vi "_RSA_PKCS1.vi"() -> ()   [LabVIEW 2023]
panel:
  out "tick":u32
  in  "Tab Control":enum32{"密钥生成", "加密解密"}(tab)
  in  "生成秘钥":bool
  in  "填入密钥":bool
  out "公钥":string
  out "私钥":string
  out "?":string
  in  "密钥位数":string(combo)="308"
  in  "原文":string="天空有着多少颗的星辰\n地上就有多少段的人生\n外头无论多么样的寒冷\n蜂蜜酒能把我们给捂热\n欢迎各位光临星河旅馆！"
  out "密文":string
  in  "密文":string
  out "原文":string
  in  "加密":bool
  in  "解密":bool
  in  "公钥":string="-----BEGIN RSA PUBLIC KEY-----\nMIIBCgKCAQECJTwZ2lRcKrdTU5zbP4z6rGr57lWznUWXeU/0eLCZ14Efdue8kDYj\ncuNkpjTIbWBGzZMtdoRwx8lVMC5QrfBdp8Z0nIlqdQvrehlQ/IY9xlbD70XQugy0\nvE1Zmccf/ex+oCsI7Rl1+JaAEsmBIPdWX6dpDelnwkPRapSc2BAyo8R3d6naFasE\nK+y4iqP5SAZjpi9/uEQ9JqqLm8QMkNIqmiqWLyoRZkTEwvw76ODYCu/k+xfulWsh\nC2aG7vTpwTCx7sU7E38QPgA/ICCj2U98wi4VcYiLVVyEXuDKF5WR4FKpMV93n8rY\nw8Kw5xqqdEjMKdE0ARgj7lb3hH9wmUEYlQIDAQAB\n-----END RSA PUBLIC KEY-----"
  in  "私钥":string="-----BEGIN RSA PRIVATE KEY-----\nMIIEpgIBAAKCAQECJTwZ2lRcKrdTU5zbP4z6rGr57lWznUWXeU/0eLCZ14Efdue8\nkDYjcuNkpjTIbWBGzZMtdoRwx8lVMC5QrfBdp8Z0nIlqdQvrehlQ/IY9xlbD70XQ\nugy0vE1Zmccf/ex+oCsI7Rl1+JaAEsmBIPdWX6dpDelnwkPRapSc2BAyo8R3d6na\nFasEK+y4iqP5SAZjpi9/uEQ9JqqLm8QMkNIqmiqWLyoRZkTEwvw76ODYCu/k+xfu\nlWshC2aG7vTpwTCx7sU7E38QPgA/ICCj2U98wi4VcYiLVVyEXuDKF5WR4FKpMV93\nn8rYw8Kw5xqqdEjMKdE0ARgj7lb3hH9wmUEYlQIDAQABAoIBAQIBlYDLU2VYIFOP\n9TZj582kGuiZQJSTtTaenvCJRwKkrT6h7rK525YsYYyFiwf8lzG+HClAETpw58h8\nJGMXM5QwRfhXRHxC9SF97Fx5toHfjNTtUsiKoUUEbAQkMzqsNFB4L6XKKKvTB9C9\nQKY6EG85RQ+MjbyTwNz7n/pGZGcmDlPM7dlFwKN5LxS931CcjIC8FcXqCb2hfPIn\nR7L4hmbvT8vSZe3LfwSMcIu3dbL7Uh1N1URtDSiFu785GYtl2WLHTrTE2F38ygYe\nY7KJ5kLNr91ULJfUatukeSolfndqnlWPisoshtopYisDeL+2olHjvl0VGk8j1t5c\nU6PAL3fhAoGBBAq9XeIIIMu9gYEY4rCES++Y1u+SGp/ET/e0aFEq9a5aiZdce9m/\nEaUsd+suffk3sqabG9Mb8SaNremsMpptrxtwVnaLlr6OZxQV2KaT+3AFI1m8Vs6d\n8IFQdD5/62XIXVCRQgUJyZwxcHY6uNZ5KwLpQ7VgTNLWFys3PnP9/wVdAoGBAIfi\nMAnVVHpeAgXo3hOd5/1FapFC0yH2tJv7VcHjd9r++0JC2xCEnLJ4P1jHHOK0sJ+W\nCHRXiY2q6ihiMtue3LbE8KQTJ4gECf6LqrEdijw8KwyQclCOhdtdtOG31gfQIlxH\n+L8lnha2Gln2kYuIHS/EnTb2v+2nCf9LM+lNwDSZAoGBAsbeEgGXU/Ck4LOwRQy/\n1utkNUWhOmlIlSe36XLZ8K83xA8Ymn2dpqGzSy9nYWQ1v6Z2KUd/iszRyQkgJCOz\n9vkC1GPcwlNnwakq2QyX3cW3wfGEUp7gIrq0aygE+dOTM4iGQrTzZG7KCFkxPosZ\n81KsrreM0TqHmqM18NH/TZSBAoGBAIYOCJR66Ne8DMTlwsmZm/hK1mKuiXrVV8MW\nxrj8fw8HRLxPFq2KFskfRmeAMCgcWK9oJbkZbzPbLR1gG4p9hIOvcTR9TR+r1GxS\nP7hySyE3vsSrcIu2v6n2HXAdnEKi/HML8gQpyXfgecjNLzN3ukuY7fz+m8SKaZt6\nBqGhOgDpAoGBAw/yVr0DlLIgLzbeIWyrIeXSE8C7c/wH1fnUlt+sILGcUZIdUR9H\nLNTdImxRtSZFOgwS7V2hT3S6X4+SavwKWLRs0Bq1ZbHVCBsx7WotmtYb8MPyJChP\nkkSuCOkYuEU5yGVSwSNHa2QpbnpoM2wGuaBAD3qGTQ4EoO4vr/4kEJqZ\n-----END RSA PRIVATE KEY-----"
  in  "填入密文":bool
  out "加解密提示":string
  in  "填入密钥":bool
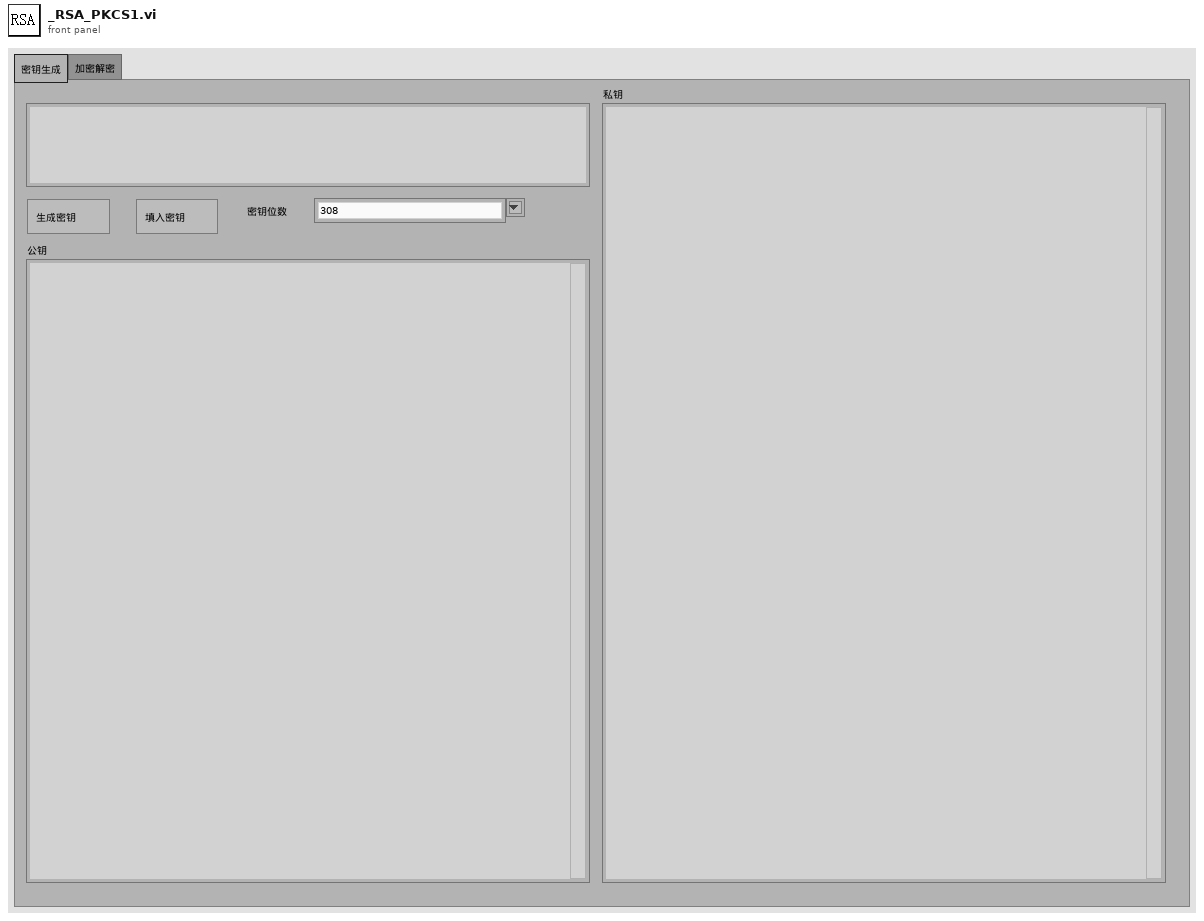
[diagram p1: front panel]
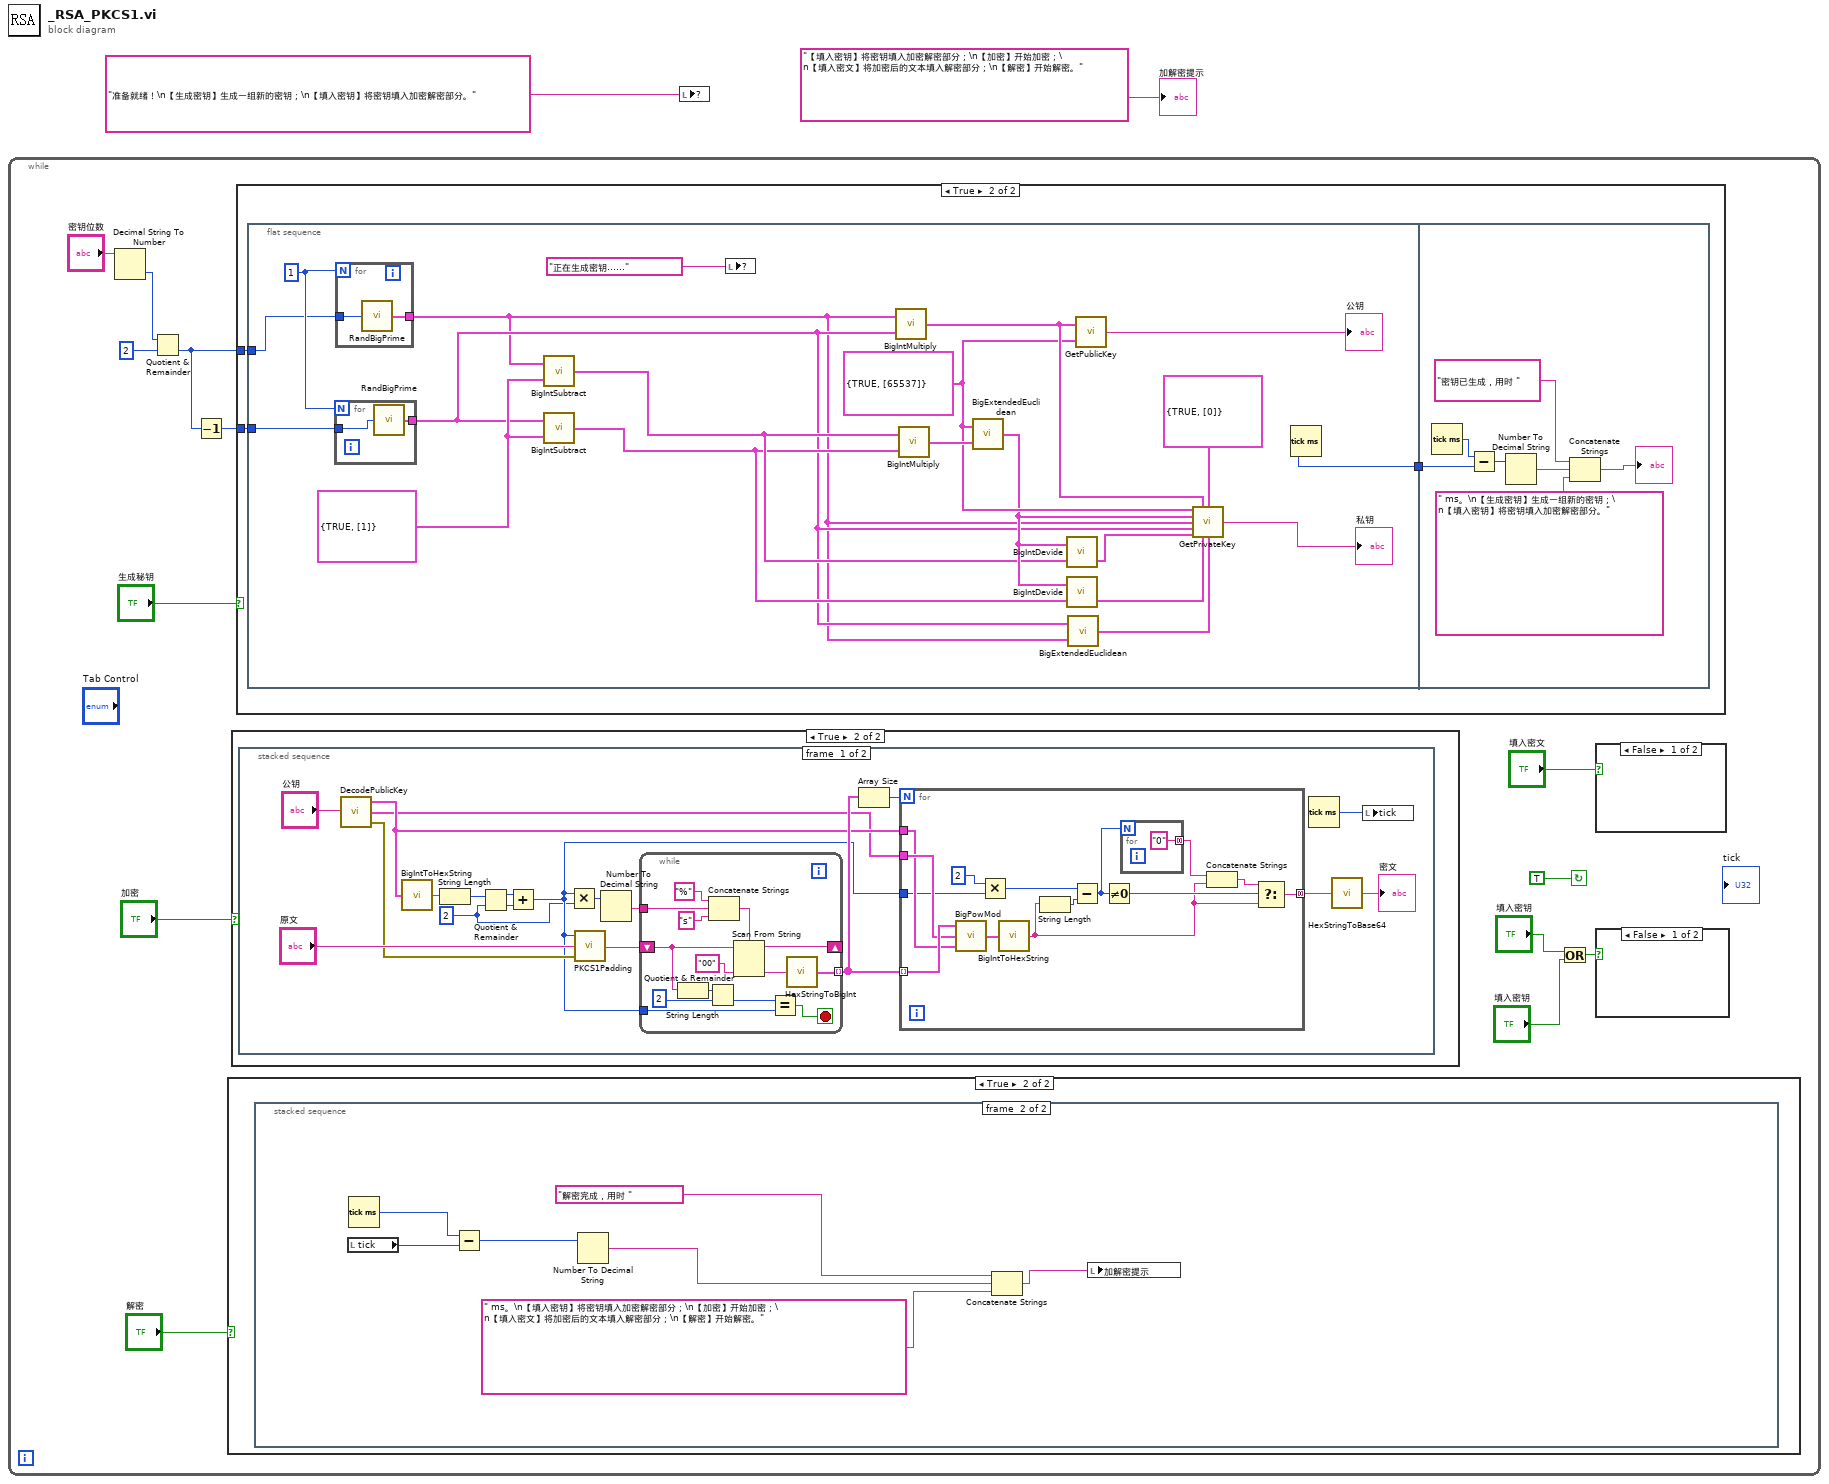
[diagram p0: block diagram]
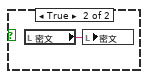
[diagram p2: hidden frame]
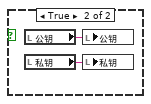
[diagram p3: hidden frame]
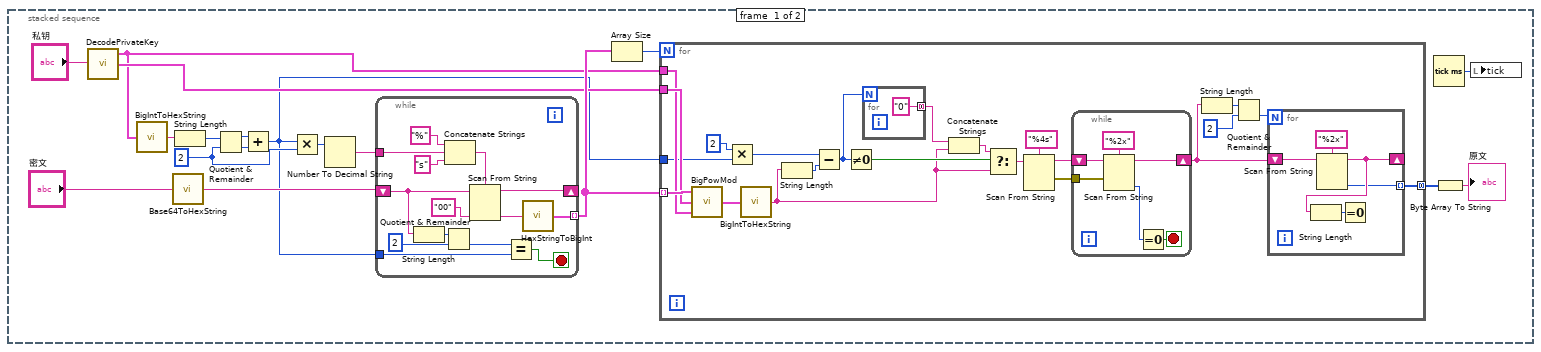
[diagram p5: hidden frame]
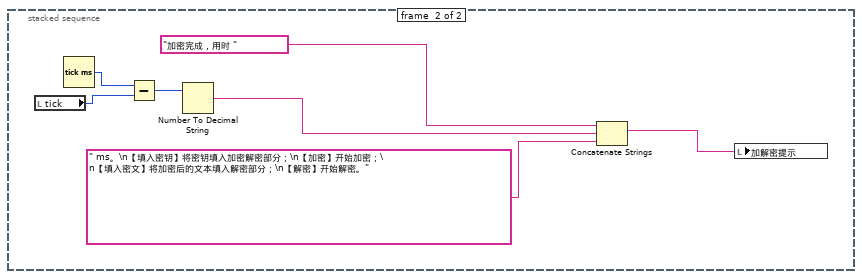
[diagram p7: hidden frame]
diagram:
  n1 = while {
    stop <- TRUE continue-if-true
    n2 = Decimal String To Number(string="密钥位数") -> (number=w8:i32)  [unwired: 2 in, 1 out]
    n3 = Quotient & Remainder(x=w8, y=2) -> (floor(x/y)=w7:i32)  [unwired: 1 out]
    n4 = Decrement(x=w7) -> (x-1=w6:i32)
    n5 = case shown="True" "解密" {
      frame False {
      }
      frame True {
        n6 = stacked-sequence {
          frame #0 {
            w31 = 2
            n7 = call "DecodePrivateKey.vi"("Private Key"="私钥") -> ("d"=w24:cluster{"P/N":bool, "Array":u64[]}, "n"=w23:cluster{"P/N":bool, "Array":u64[]})  [unwired: 2 in, 1 out]
            n8 = call "BigIntToHexString.vi"("a"=w23) -> ("Hex string"=w35:string)
            n9 = call "Base64ToHexString.vi"("BASE64 string"="密文") -> ("Hex"=w27:string)
            n10 = String Length(string=w35) -> (length=w34:i32)
            n11 = Quotient & Remainder(x=w34, y=w31) -> (x-y*floor(x/y)=w33:i32, floor(x/y)=w32:i32)
            n12 = Add(x=w33, y=w32) -> (x+y=w22:i32)
            n13 = Multiply(x=w22, y=w31) -> (x*y=w30:i32)
            n14 = Number To Decimal String(number=w30) -> (decimal integer string=w29:string)  [unwired: 1 in]
            n15 = while {
              tunnel: w29 -> [w83]
              tunnel: w22 -> [w78]
              shift-right: [w75] -> _
              shift-left: w27 -> [w77]
              tunnel: [w74] -> w25 mode=indexing
              stop <- w76 stop-if-true
              n16 = String Length(string=w77) -> (length=w72:i32)
              n17 = Quotient & Remainder(x=w72, y=2) -> (floor(x/y)=w73:i32)  [unwired: 1 out]
              n18 = Concatenate Strings("%", w83, "s") -> (w81:string)
              n19 = Scan From String(format string=w81, input string=w77, default 1="00") -> (remaining string=w75:string, output 1=w79:string)  [unwired: 2 in, 2 out]
              n20 = Equal?(x=w73, y=w78) -> (x = y?=w76:bool)
              n21 = call "HexStringToBigInt.vi"("String (hex)"=w79) -> ("Int"=w74:cluster{"P/N":bool, "Array":u64[]})
            }
            n22 = Array Size(array=w25) -> (size(s)=w26:i32)
            n23 = for {
              N: w26 -> [_]
              tunnel: w25 -> [w58] mode=indexing
              tunnel: w24 -> [w57]
              tunnel: w23 -> [w56]
              tunnel: w22 -> [w43]
              tunnel: [w41] -> w21 mode=concatenating
              n24 = call "BigPowMod.vi"("c"=w56, "b"=w57, "a"=w58) -> ("a ^ b mod c"=w49:cluster{"Boolean":bool, "Array":u64[]})
              n25 = Multiply(x=2, y=w43) -> (x*y=w47:i32)
              n26 = call "BigIntToHexString.vi"("a"=w49) -> ("Hex string"=w51:string)
              n27 = String Length(string=w51) -> (length=w55:i32)
              n28 = Subtract(x=w47, y=w55) -> (x-y=w53:i32)
              n29 = Not Equal To 0?(x=w53) -> (x != 0?=w54:bool)
              n30 = for {
                N: w53 -> [_]
                tunnel: ["0"] -> w52 mode=concatenating
              }
              n31 = Concatenate Strings(w52, w51) -> (w50:string)
              n32 = Select(t=w50, s=w54, f=w51) -> (s? t:f=w46:string)
              n33 = Scan From String(format string="%4s", input string=w46) -> (remaining string=w42:string, error out=w44:errorcluster)  [unwired: 4 in, 1 out]
              n34 = while {
                tunnel: w44 -> [w69]
                shift-right: [w64] -> w40
                shift-left: w42 -> [w65]
                stop <- w66 stop-if-true
                n35 = Scan From String(format string="%2x", input string=w65, error in=w69) -> (remaining string=w64:string, output 1=w67:u32)  [unwired: 2 in, 2 out]
                n36 = Equal To 0?(x=w67) -> (x = 0?=w66:bool)
              }
              n37 = String Length(string=w40) -> (length=w38:i32)
              n38 = Quotient & Remainder(x=w38, y=2) -> (floor(x/y)=w39:i32)  [unwired: 1 out]
              n39 = for {
                N: w39 -> [_]
                shift-right: [w61] -> _
                shift-left: w40 -> [w62]
                tunnel: [w59] -> w41 mode=indexing
                n40 = Scan From String(format string="%2x", input string=w62) -> (remaining string=w61:string, output 1=w59:u32)  [unwired: 3 in, 2 out]
                n41 = String Length(string=w61) -> (length=w60:i32)
                n42 = Equal To 0?(x=w60) -> ()  [unwired: 1 out]
              }
            }
            n43 = Tick Count (ms)() -> (millisecond timer value=w19:u32)
            n44 = Byte Array To String(unsigned byte array=w21) -> (string=→"原文":string)
            n45 = local write "tick"(w19) -> ()
          }
          frame #1 {
            n46 = local read "tick"() -> (w85:u32)
            n47 = Tick Count (ms)() -> (millisecond timer value=w86:u32)
            n48 = Subtract(x=w86, y=w85) -> (x-y=w91:u32)
            n49 = Number To Decimal String(number=w91) -> (decimal integer string=w89:string)  [unwired: 1 in]
            n50 = Concatenate Strings("解密完成，用时 ", w89, " ms。\n【填入密钥】将密钥填入加密解密部分；\n【加密】开始加密；\n【填入密文】将加密后的文本填入解密部分；\n【解密】开始解密。") -> (w87:string)
            n51 = local write "加解密提示"(w87) -> ()
          }
        }
      }
    }
    n52 = case shown="True" "加密" {
      frame False {
      }
      frame True {
        n53 = stacked-sequence {
          frame #0 {
            w93 = 2
            n54 = call "DecodePublicKey.vi"("Public Key"="公钥") -> ("error out"=w104:errorcluster, "e"=w98:cluster{"P/N":bool, "Array":u64[]}, "n"=w99:cluster{"P/N":bool, "Array":u64[]})  [unwired: 2 in]
            n55 = call "BigIntToHexString.vi"("a"=w99) -> ("Hex string"=w108:string)
            n56 = String Length(string=w108) -> (length=w107:i32)
            n57 = Quotient & Remainder(x=w107, y=w93) -> (x-y*floor(x/y)=w106:i32, floor(x/y)=w105:i32)
            n58 = Add(x=w106, y=w105) -> (x+y=w97:i32)
            n59 = Multiply(x=w97, y=w93) -> (x*y=w94:i32)
            n60 = call "PKCS1Padding.vi"("error in (no error)"=w104, "Message"="原文", "Length"=w97) -> ("Hex (After Padding)"=w103:string)  [unwired: 1 in, 1 out]
            n61 = Number To Decimal String(number=w94) -> (decimal integer string=w102:string)  [unwired: 1 in]
            n62 = while {
              tunnel: w102 -> [w138]
              tunnel: w97 -> [w133]
              shift-right: [w130] -> _
              shift-left: w103 -> [w132]
              tunnel: [w129] -> w100 mode=indexing
              stop <- w131 stop-if-true
              n63 = String Length(string=w132) -> (length=w127:i32)
              n64 = Quotient & Remainder(x=w127, y=2) -> (floor(x/y)=w128:i32)  [unwired: 1 out]
              n65 = Concatenate Strings("%", w138, "s") -> (w136:string)
              n66 = Scan From String(format string=w136, input string=w132, default 1="00") -> (remaining string=w130:string, output 1=w134:string)  [unwired: 2 in, 2 out]
              n67 = Equal?(x=w128, y=w133) -> (x = y?=w131:bool)
              n68 = call "HexStringToBigInt.vi"("String (hex)"=w134) -> ("Int"=w129:cluster{"P/N":bool, "Array":u64[]})
            }
            n69 = Array Size(array=w100) -> (size(s)=w101:i32)
            n70 = for {
              N: w101 -> [_]
              tunnel: w100 -> [w124] mode=indexing
              tunnel: w99 -> [w122]
              tunnel: w98 -> [w123]
              tunnel: w97 -> [w113]
              tunnel: [w117] -> w95 mode=concatenating
              n71 = call "BigPowMod.vi"("c"=w122, "b"=w123, "a"=w124) -> ("a ^ b mod c"=w121:cluster{"Boolean":bool, "Array":u64[]})
              n72 = Multiply(x=2, y=w113) -> (x*y=w115:i32)
              n73 = call "BigIntToHexString.vi"("a"=w121) -> ("Hex string"=w112:string)
              n74 = String Length(string=w112) -> (length=w120:i32)
              n75 = Subtract(x=w115, y=w120) -> (x-y=w118:i32)
              n76 = Not Equal To 0?(x=w118) -> (x != 0?=w119:bool)
              n77 = for {
                N: w118 -> [_]
                tunnel: ["0"] -> w116 mode=concatenating
              }
              n78 = Concatenate Strings(w116, w112) -> (w111:string)
              n79 = Select(t=w111, s=w119, f=w112) -> (s? t:f=w117:string)
            }
            n80 = Tick Count (ms)() -> (millisecond timer value=w92:u32)
            n81 = call "HexStringToBase64.vi"("Hex"=w95) -> ("BASE64 string"=→"密文":string)
            n82 = local write "tick"(w92) -> ()
          }
          frame #1 {
            n83 = local read "tick"() -> (w140:u32)
            n84 = Tick Count (ms)() -> (millisecond timer value=w141:u32)
            n85 = Subtract(x=w141, y=w140) -> (x-y=w146:u32)
            n86 = Number To Decimal String(number=w146) -> (decimal integer string=w144:string)  [unwired: 1 in]
            n87 = Concatenate Strings("加密完成，用时 ", w144, " ms。\n【填入密钥】将密钥填入加密解密部分；\n【加密】开始加密；\n【填入密文】将加密后的文本填入解密部分；\n【解密】开始解密。") -> (w142:string)
            n88 = local write "加解密提示"(w142) -> ()
          }
        }
      }
    }
    n89 = case shown="True" "生成秘钥" {
      tunnel: w7 -> [_ w147]
      tunnel: w6 -> [_ w148]
      frame False {
      }
      frame True {
        n90 = flat-sequence {
          tunnel: [w168] -> w149
          tunnel: w147 -> [w165]
          tunnel: w148 -> [w164]
          tunnel: w149 -> [w179]
          frame #0 {
            w158 = cluster{bool, u64[]} {TRUE, [65537]}
            w167 = 1
            w169 = cluster{bool, u64[]} {TRUE, [1]}
            n91 = for {
              N: w167 -> [_]
              tunnel: [w171] -> w152
              tunnel: w164 -> [w170]
              n92 = call "RandBigPrime.vi"("Numeric"=w170) -> ("Random Prime (1e18)"=w171:cluster{"Boolean":bool, "Array":u64[]})
            }
            n93 = for {
              N: w167 -> [_]
              tunnel: [w173] -> w151
              tunnel: w165 -> [w172]
              n94 = call "RandBigPrime.vi"("Numeric"=w172) -> ("Random Prime (1e18)"=w173:cluster{"Boolean":bool, "Array":u64[]})
            }
            n95 = call "BigIntSubtract.vi"("b"=w169, "a"=w151) -> ("a - b"=w156:cluster{"Boolean":bool, "Array":u64[]})
            n96 = call "BigIntSubtract.vi"("b"=w169, "a"=w152) -> ("a - b"=w155:cluster{"Boolean":bool, "Array":u64[]})
            n97 = local write item#13("正在生成密钥……") -> ()
            n98 = call "BigIntMultiply.vi"("b"=w152, "a"=w151) -> ("a * b"=w159:cluster{"Boolean":bool, "Array":u64[]})
            n99 = call "BigIntMultiply.vi"("b"=w155, "a"=w156) -> ("a * b"=w163:cluster{"Boolean":bool, "Array":u64[]})
            n100 = call "BigExtendedEuclidean.vi"("b"=w163, "a"=w158) -> ("c (ac mod(b) = 1)"=w157:cluster{"Boolean":bool, "Array":u64[]})
            n101 = call "BigIntDevide.vi"("b"=w156, "a"=w157) -> ("a % b"=w154:cluster{"Boolean":bool, "Array":u64[]})  [unwired: 1 out]
            n102 = call "BigIntDevide.vi"("b"=w155, "a"=w157) -> ("a % b"=w153:cluster{"Boolean":bool, "Array":u64[]})  [unwired: 1 out]
            n103 = call "BigExtendedEuclidean.vi"("b"=w151, "a"=w152) -> ("c (ac mod(b) = 1)"=w150:cluster{"Boolean":bool, "Array":u64[]})
            n104 = call "GetPublicKey.vi"("e"=w158, "n"=w159) -> ("Public Key"=→"公钥":string)
            n105 = call "GetPrivateKey.vi"("e"=w158, "n"=w159, "Version"=cluster{bool, u64[]} {TRUE, [0]}, "d"=w157, "p"=w151, "q"=w152, "d mod(p - 1)"=w154, "d mod(q - 1)"=w153, "q^-1 mod(p)"=w150) -> ("Public Key"=→"私钥":string)  [unwired: 6 in]
            n106 = Tick Count (ms)() -> (millisecond timer value=w168:u32)
          }
          frame #1 {
            n107 = Tick Count (ms)() -> (millisecond timer value=w180:u32)
            n108 = Subtract(x=w180, y=w179) -> (x-y=w178:u32)
            n109 = Number To Decimal String(number=w178) -> (decimal integer string=w176:string)  [unwired: 1 in]
            n110 = Concatenate Strings("密钥已生成，用时 ", w176, " ms。\n【生成密钥】生成一组新的密钥；\n【填入密钥】将密钥填入加密解密部分。") -> (→"?":string)
          }
        }
      }
    }
    n111 = Or(x="填入密钥", y="填入密钥") -> (x .or. y?=w5:bool)
    n112 = case shown="False" "填入密文" {
      frame False {
      }
      frame True {
        n113 = local read "密文"() -> (w16:string)
        n114 = local write "密文"(w16) -> ()
      }
    }
    n115 = case shown="False" w5 {
      frame False {
      }
      frame True {
        n116 = local read "公钥"() -> (w18:string)
        n117 = local read "私钥"() -> (w17:string)
        n118 = local write "公钥"(w18) -> ()
        n119 = local write "私钥"(w17) -> ()
      }
    }
  }
  n120 = local write item#13("准备就绪！\n【生成密钥】生成一组新的密钥；\n【填入密钥】将密钥填入加密解密部分。") -> ()
  "加解密提示" <- "【填入密钥】将密钥填入加密解密部分；\n【加密】开始加密；\n【填入密文】将加密后的文本填入解密部分；\n【解密】开始解密。"
